vi "Calc - PODF.vi"(11 "00-00-9220":dbl[](array[numeric])) -> (3 "PODF":dbl)   [LabVIEW 2018, in "Controller (Host).lvlib"]
uses:
  Controller (Host).lvlib
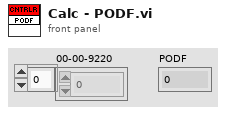
[diagram p1: front panel]
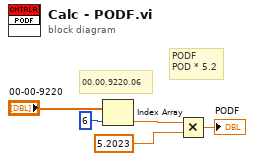
[diagram p0: block diagram]
diagram:
  # "00.00.9220.06"
  # "PODF\nPOD * 5.2"
  n1 = Index Array(array="00-00-9220", index=6) -> (element=w3:dbl)
  n2 = Multiply(x=w3, y=5.2023) -> (x*y=→"PODF":dbl)
